vi "AIT 429 Label Page.vi"(8 "error in (no error)":errorcluster, 11 "Node Ptr":T3 format="%.0x") -> (0 "error out":errorcluster)   [LabVIEW 2015, in "AIT 429 System Explorer.lvlib"]
uses:
  AIT 429 System Explorer.lvlib
  <vilib>/NI Veristand/Custom Device API/Custom Device Item Ref.ctl
  Shared/Controls and Global/Label.ctl
  Shared/Controls and Global/TransferType.ctl
  Shared/Controls and Global/Global.vi
  <vilib>/NI Veristand/Custom Device API/Get Item Property (Variant).vi
  <vilib>/NI Veristand/Custom Device API/Get Item Property (Double).vi
  <vilib>/NI Veristand/Custom Device API/Get Item Property (U32).vi
  <vilib>/NI Veristand/Custom Device API/Get Item Property (Boolean).vi
  <vilib>/NI Veristand/Custom Device API/Custom Device API.lvlib
  Shared/AIT 429 Shared.lvlib
panel:
  out "TransferType":T1
  out "SDI":T2 format="%.0o"
  out "SDI Enabled":bool
  out "Transfer Rate (Hz)":dbl
  out "Label":T2 format="%.0o"
  in  "Header":cluster{"Section Name":string}={"Section Name"="AIT 429 Label"}
  in  "Description":string
  out "Name":string
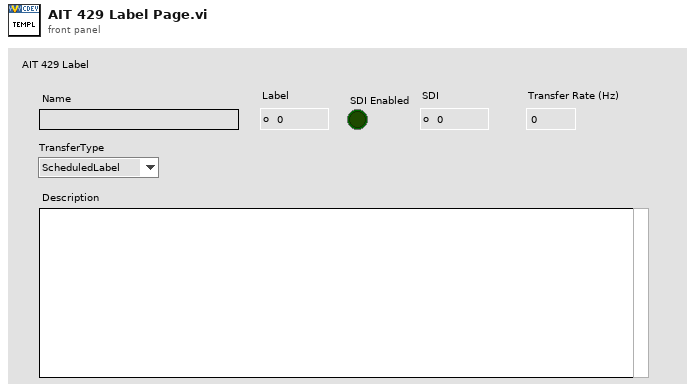
[diagram p1: front panel]
types:
  T1 = typedef "AIT 429 Shared.lvlib/TransferType.ctl" = enum16{"ScheduledLabel", "Acyclic", "Block", "Strobe"}
  T2 = typedef "AIT 429 Shared.lvlib/Label.ctl" = u8
  T3 = typedef "Custom Device API.lvlib/Custom Device Item Ref.ctl" = u64
  T4 = typedef "Custom Device API.lvlib/Custom Device Item Info.ctl" = cluster{"Name":string, "Is Channel":bool, "GUID":string, "Is Waveform":bool}
  T5 = typedef "Custom Device API.lvlib/Custom Device Commands.ctl" = enum16{"Default", "Item renamed", "Shutdown", "Dynamic button pressed"}
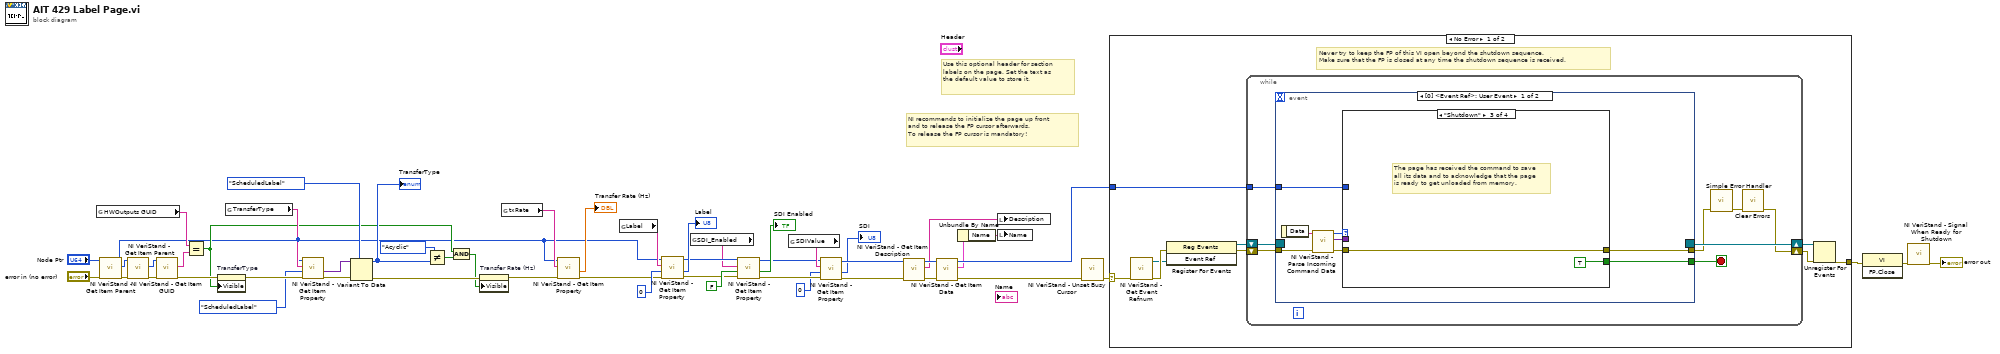
[diagram p0: block diagram]
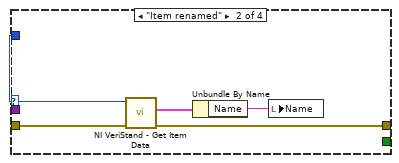
[diagram p3: hidden frame]
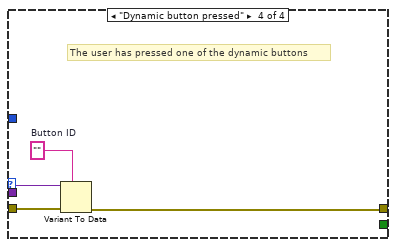
[diagram p4: hidden frame]
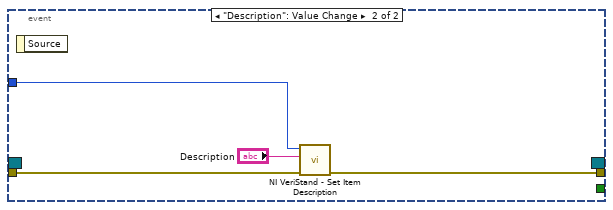
[diagram p5: hidden frame]
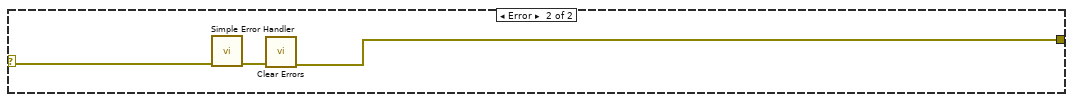
[diagram p6: hidden frame]
diagram:
  # "Use this optional header for section labels on the page. Set the text as the default value to store it."
  # "NI recommends to initialize the page up front\nand to release the FP cursor afterwards.\nTo release the FP cursor is mandatory!"
  n1 = global read "Global.vi" "HWOutputs GUID"() -> (w32:string)
  n2 = call <vilib>:"NI VeriStand - Get Item Parent.vi"("error in (no error)"="error in (no error)", "Item Ref in"="Node Ptr") -> ("error out"=w36:errorcluster, "Parent Ref"=w35:T3, "Item Ref out"=w2:T3)  [unwired: 6 in, 1 out]
  n3 = call <vilib>:"NI VeriStand - Get Item Parent.vi"("error in (no error)"=w36, "Item Ref in"=w35) -> ("error out"=w34:errorcluster, "Parent Ref"=w29:T3)  [unwired: 6 in, 2 out]
  n4 = call <vilib>:"NI VeriStand - Get Item GUID.vi"("error in (no error)"=w34, "Item Ref in"=w29) -> ("error out"=w11:errorcluster, "GUID"=w33:string)  [unwired: 7 in, 1 out]
  n5 = Equal?(x=w32, y=w33) -> (x = y?=w5:bool)
  n6 = property on="TransferType" class="Enum (strict)"(error in=w11, "Visible"=w5) -> (error out=w10:errorcluster)  [unwired: 1 in, 1 out]
  n7 = global read "Global.vi" "TransferType"() -> (w15:string)
  n8 = call-poly <vilib>:"NI VeriStand - Get Item Property.vi"("error in (no error)"=w10, "Default Value"=TransferType."ScheduledLabel" ("TransferType"), "Property Name"=w15, "Item Ref in"=w2) -> ("error out"=w14:errorcluster, "Value"=w12:variant)  [unwired: 4 in, 2 out]
  n9 = Variant To Data(error in=w14, type=TransferType."ScheduledLabel" ("TransferType"), Variant=w12) -> (data=w8:T1, error out=w9:errorcluster)
  "TransferType" <- w8
  n10 = Not Equal?(x=TransferType."Acyclic", y=w8) -> (x != y?=w6:bool)
  n11 = And(x=w5, y=w6) -> (x .and. y?=w4:bool)
  n12 = property on="Transfer Rate (Hz)" class="DigNum (strict)"(error in=w9, "Visible"=w4) -> (error out=w31:errorcluster)  [unwired: 1 in, 1 out]
  n13 = global read "Global.vi" "txRate"() -> (w40:string)
  n14 = call-poly <vilib>:"NI VeriStand - Get Item Property.vi"("error in (no error)"=w31, "Property Name"=w40, "Item Ref in"=w2) -> ("error out"=w3:errorcluster, "Value"=→"Transfer Rate (Hz)":dbl)  [unwired: 5 in, 2 out]
  n15 = global read "Global.vi" "Label"() -> (w41:string)
  n16 = call-poly <vilib>:"NI VeriStand - Get Item Property.vi"("error in (no error)"=w3, "Default Value"=T2 0 ("Label"), "Property Name"=w41, "Item Ref in"=w2) -> ("error out"=w22:errorcluster, "Value"=→"Label":u32, "Item Ref out"=w27:T3)  [unwired: 4 in, 1 out]
  n17 = global read "Global.vi" "SDI_Enabled"() -> (w26:string)
  n18 = call-poly <vilib>:"NI VeriStand - Get Item Property.vi"("error in (no error)"=w22, "Default Value"=FALSE, "Property Name"=w26, "Item Ref in"=w27) -> ("error out"=w21:errorcluster, "Value"=→"SDI Enabled":bool, "Item Ref out"=w19:T3)  [unwired: 4 in, 1 out]
  n19 = global read "Global.vi" "SDIValue"() -> (w23:string)
  n20 = call-poly <vilib>:"NI VeriStand - Get Item Property.vi"("error in (no error)"=w21, "Default Value"=T2 0 ("Label"), "Property Name"=w23, "Item Ref in"=w19) -> ("error out"=w20:errorcluster, "Value"=→"SDI":u32, "Item Ref out"=w18:T3)  [unwired: 4 in, 1 out]
  n21 = call <vilib>:"NI VeriStand - Get Item Description.vi"("error in (no error)"=w20, "Item Ref in"=w18) -> ("error out"=w44:errorcluster, "Description"=w45:string, "Item Ref out"=w46:T3)  [unwired: 7 out]
  n22 = call <vilib>:"NI VeriStand - Get Item Data.vi"("error in (no error)"=w44, "Item Ref in"=w46) -> ("error out"=w49:errorcluster, "Item Info"=w43:T4, "Item Ref out"=w47:T3)  [unwired: 7 out]
  n23 = Unbundle By Name(w43) -> ("Name"=w42:string)
  n24 = local write "Description"(w45) -> ()
  n25 = local write "Name"(w42) -> ()
  n26 = call <vilib>:"NI VeriStand - Unset Busy Cursor.vi"("error in (no error)"=w49) -> ("error out"=w48:errorcluster)  [unwired: 10 out]
  n27 = case shown="No Error" w48 {
    selector: w48 -> [w53 w96]
    tunnel: [w58 w94] -> w52
    tunnel: w47 -> [w54 _]
    frame No Error {
      # "Never try to keep the FP of this VI open beyond the shutdown sequence.\nMake sure that the FP is closed at any time the shutdown sequence is received."
      n28 = call <vilib>:"NI VeriStand - Get Event Refnum.vi"("error in (no error)"=w53) -> ("error out"=w61:errorcluster, "Event Ref"=w57:refnum<user-event>)  [unwired: 9 out]
      n29 = register-events(error in=w61, w57) -> (reference out=w55:refnum<event-registration>, error out=w56:errorcluster)  [unwired: 1 in]
      n30 = while {
        tunnel: w54 -> [w65]
        shift-right: [w62] -> w59
        shift-left: w56 -> [w68]
        shift-right: [w69] -> w60
        shift-left: w55 -> [w67]
        stop <- w66 stop-if-true
        n31 = event shown="[0] <Event Ref>: User Event" {
          selector: w67 -> [_ _]
          dyn-events: [_ _] -> w69
          timeout: _ -> [_ _]
          tunnel: w68 -> [w77 w92]
          tunnel: [w73 _] -> w66
          tunnel: [w72 w91] -> w64
          tunnel: w65 -> [w71 w93]
          event User Event {
            n32 = event-data() -> ("Data"=w76:string)  [unwired: 1 out]
            n33 = call <vilib>:"NI VeriStand - Parse Incoming Command Data.vi"("error in (no error)"=w77, "Incoming data"=w76) -> ("error out"=w75:errorcluster, "Outgoing data"=w70:variant, "Action"=w74:T5)  [unwired: 7 out]
            n34 = case shown="\"Shutdown\"" w74 {
              tunnel: w75 -> [w78 w83 w84 w89]
              tunnel: [_ _ TRUE _] -> w73
              tunnel: [w78 w80 w84 w86] -> w72
              tunnel: w71 -> [_ w82 _ _]
              tunnel: w70 -> [_ _ _ w88]
              frame "Default", Default {
              }
              frame "Item renamed" {
                n35 = call <vilib>:"NI VeriStand - Get Item Data.vi"("error in (no error)"=w83, "Item Ref in"=w82) -> ("error out"=w80:errorcluster, "Item Info"=w81:T4)  [unwired: 8 out]
                n36 = Unbundle By Name(w81) -> ("Name"=w79:string)
                n37 = local write "Name"(w79) -> ()
              }
              frame "Shutdown" {
                # "The page has received the command to save all its data and to acknowledge that the page is ready to get unloaded from memory."
              }
              frame "Dynamic button pressed" {
                w87 = ""  # Button ID
                # "The user has pressed one of the dynamic buttons"
                n38 = Variant To Data(error in=w89, type=w87, Variant=w88) -> (error out=w86:errorcluster)  [unwired: 1 out]
              }
            }
          }
          event "Description": Value Change {
            n39 = event-data() -> ()  [unwired: 2 out]
            n40 = call <vilib>:"NI VeriStand - Set Item Description.vi"("error in (no error)"=w92, "Description"="Description", "Item Ref in"=w93) -> ("error out"=w91:errorcluster)  [unwired: 8 out]
          }
        }
        n41 = call <vilib>:"Simple Error Handler.vi"("error in (no error)"=w64) -> ("error out"=w63:errorcluster)  [unwired: 1 in, 7 out]
        n42 = call <vilib>:"Clear Errors.vi"("error in (no error)"=w63) -> ("error out"=w62:errorcluster)  [unwired: 1 in, 5 out]
      }
      n43 = Unregister For Events(event registration refnum=w60, error in=w59) -> (error out=w58:errorcluster)
    }
    frame Error {
      n44 = call <vilib>:"Simple Error Handler.vi"("error in (no error)"=w96) -> ("error out"=w95:errorcluster)  [unwired: 1 in, 7 out]
      n45 = call <vilib>:"Clear Errors.vi"("error in (no error)"=w95) -> ("error out"=w94:errorcluster)  [unwired: 1 in, 5 out]
    }
  }
  n46 = invoke class="VI" method="FP.Close"(error in=w52) -> (error out=w51:errorcluster)  [unwired: 2 in, 2 out]
  n47 = call <vilib>:"NI VeriStand - Signal When Ready for Shutdown.vi"("error in (no error)"=w51) -> ("error out"=→"error out":errorcluster)  [unwired: 10 out]
